vi "tarea2.vi"() -> ()   [LabVIEW 2016]
panel:
  in  "D":bool
  out "Z":bool
  in  "C":bool
  out "Y":bool
  in  "B":bool
  out "X":bool
  in  "A":bool
  out "W":bool
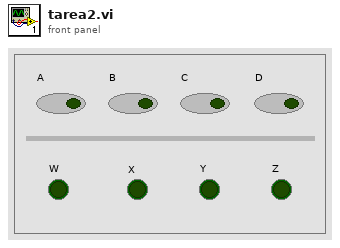
[diagram p1: front panel]
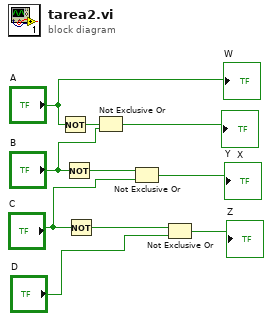
[diagram p0: block diagram]
diagram:
  n1 = Not(x="A") -> (.not. x?=w5:bool)
  n2 = Not(x="B") -> (.not. x?=w4:bool)
  n3 = Not(x="C") -> (.not. x?=w3:bool)
  n4 = Not Exclusive Or(1:"B", 2:w5) -> (0:→"X":bool)
  n5 = Not Exclusive Or(1:"C", 2:w4) -> (0:→"Y":bool)
  n6 = Not Exclusive Or(1:"D", 2:w3) -> (0:→"Z":bool)
  "W" <- "A"
